vi "PXI-Init DLL.vi"(11 "error in (no error)":errorcluster) -> (15 "error out":errorcluster)   [LabVIEW 2020]
doc: "Performs a dummy setting of the AO gains, in the process initializing the related DLLs and NI-supplied code. \n\nApparently, the operation below is slow the first time it executes, at least slow enough to cause measurement VIs (i.e. the ABR I/O controller) to lag behind in the main PXI DAQ measure loop. (Thus producing the dreaded annoying -200621 error). \n\nSo far, it appears that calling this subVI when initializing the main experiment controller is sufficient to avoid the \"startup\" error. It could also be called within each individual measurement controller.\n\nKEH 9/9/09"
uses:
  DAQ Engine VIs/AO Gain and Multiplier VIs/DAQtoVISA.dll
panel:
  # "Performs a dummy setting of the AO gains, in the process initializing the related DLLs and NI-supplied code. \n\nApparently, the operation below is slow the first time it executes, at least slow enough to cause measurement VIs (i.e. the ABR I/O controller) to lag behind in the main PXI DAQ measure loop. (Thus producing the dreaded annoying -200621 error). \n\nSo far, it appears that calling this subVI when initializing the main experiment controller is sufficient to avoid the \"startup\" error. It could also be called within each individual measurement controller.\n\nKEH 9/9/09"
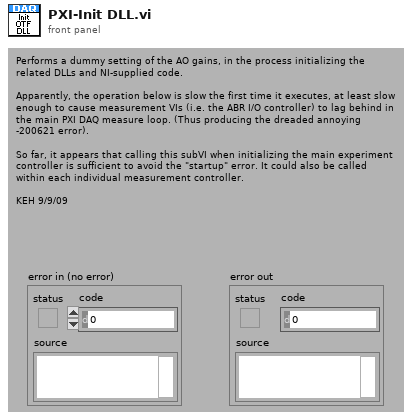
[diagram p1: front panel]
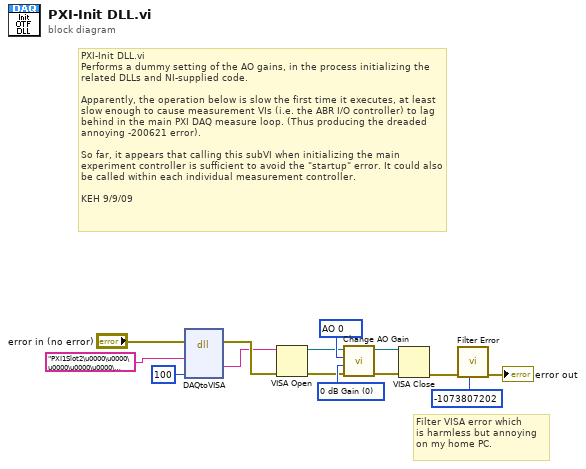
[diagram p0: block diagram]
diagram:
  w11 = u16 0 items=["0 dB Gain"=0, "20 dB Gain"=2, "40 dB Gain"=4] ("Gain Setting")
  w12 = u16 1536 items=["AO 0"=1536, "AO 1"=1540] ("AO Channel")
  # "Filter VISA error which\nis harmless but annoying\non my home PC."
  # "PXI-Init DLL.vi\nPerforms a dummy setting of the AO gains, in the process initializing the related DLLs and NI-supplied code. \n\nApparently, the operation below is slow the first time it executes, at least slow enough to cause measurement VIs (i.e. the ABR I/O controller) to lag behind in the main PXI DAQ measure loop. (Thus producing the dreaded annoying -200621 error). \n\nSo far, it appears that calling this subVI when initializing the main experiment controller is sufficient to avoid the \"startup\" error. It could also be called within each individual measurement controller.\n\nKEH 9/9/09"
  n1 = dll-call lib="D:/Experiment VIs/PXI DAQ VIs/DAQ Engine VIs/AO Gain and Multiplier VIs/DAQtoVISA.dll" fn="DAQtoVISA"(error in="error in (no error)", "DAQmxName"=tag "PXI1Slot2\u0000\u0000\u0000\u0000\u0000\u0000\u0000\u0000\u0000\u0000\u0000\u0000\u0000\u0000\u0000\u0000\u0000\u0000\u0000\u0000\u0000\u0000\u0000\u0000\u0000\u0000\u0000\u0000\u0000\u0000\u0000\u0000\u0000\u0000\u0000\u0000\u0000\u0000\u0000\u0000\u0000\u0000\u0000\u0000\u0000\u0000\u0000\u0000\u0000\u0000\u0000\u0000\u0000\u0000\u0000\u0000\u0000\u0000\u0000\u0000\u0000\u0000\u0000\u0000\u0000\u0000\u0000\u0000\u0000\u0000\u0000\u0000\u0000\u0000\u0000\u0000\u0000\u0000\u0000\u0000\u0000\u0000\u0000\u0000\u0000\u0000\u0000\u0000\u0000\u0000\u0000" ("element"), "len"=100) -> (error out=w9:errorcluster, "VISAName"=w8:string)  [unwired: 6 in, 1 out]
  n2 = VISA Open(error in (no error)=w9, VISA resource name=w8) -> (VISA resource name=w7:refnum<visa-resource-name>, error out=w10:errorcluster)  [unwired: 3 in]
  n3 = call "Change AO Gain.vi"("error in"=w10, "Gain Setting"=w11, "AO Channel"=w12, "VISA resource name 2"=w7) -> ("error out"=w6:errorcluster, "VISA resource name"=w5:refnum<visa-resource-name>)  [unwired: 4 in]
  n4 = VISA Close(VISA resource name=w5, error in (no error)=w6) -> (error out=w3:errorcluster)
  n5 = call "Filter Error.vi"("error in (no error)"=w3, "code to ignore"=-1073807202) -> ("error out"=→"error out":errorcluster)  [unwired: 9 in]
